vi "Ann_int.vi"(0 "Data":dbl[](array[numeric]), 1 "Loss Function":enum16{"MSE", "MAE"}(ring), 2 "Regularization":T1, 5 "Target":dbl format="%#_13g", 7 "Training?":bool, 9 "Parameters":T3, 13 "Adam Data In":T2) -> (4 "Output":dbl, 6 "Error":dbl, 10 "Adjusted Parameters":T3, 14 "Adam Data Out":T2)   [LabVIEW 2018]
uses:
  Adam_data.ctl
  Globals.vi
  Layer.vi
  Layer1d.vi
panel:
  out "Error Codes":i32[](array[numeric])
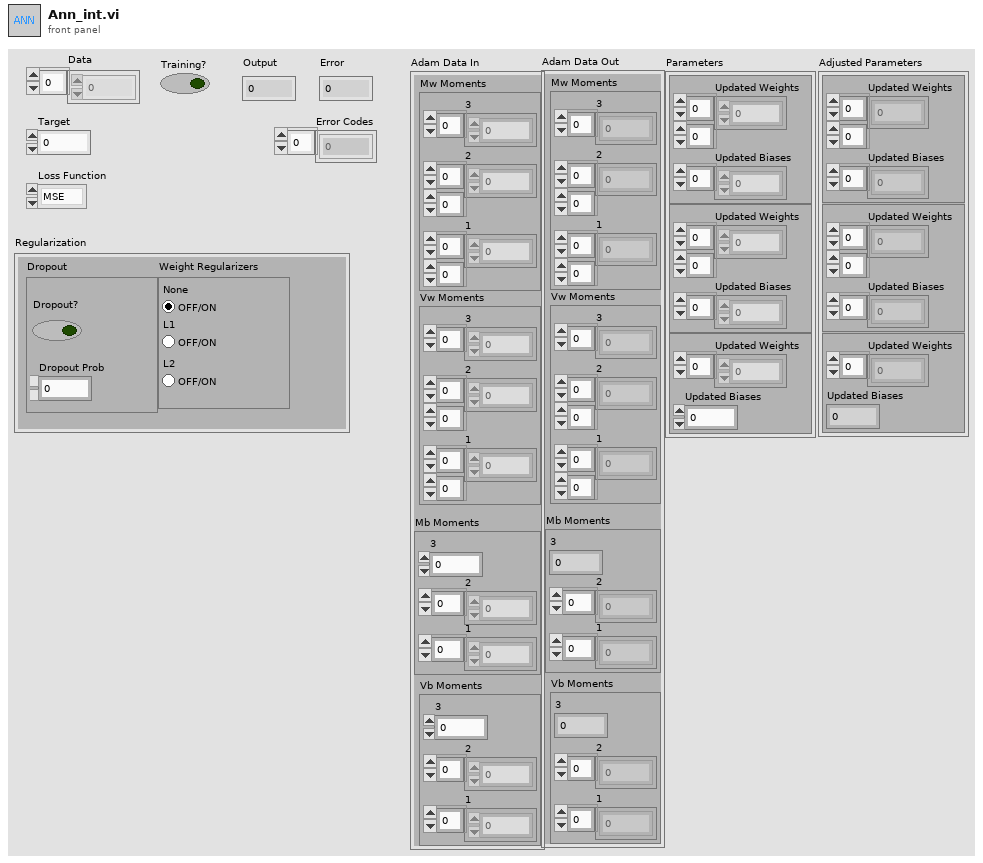
[diagram p1: front panel]
types:
  T1 = cluster{"Dropout":cluster{"Dropout?":bool, "Dropout Prob":dbl}, "Weight Regularizers":enum32{"None", "L1", "L2"}}
  T2 = typedef "Adam_data.ctl" = cluster{"Mw Moments":cluster{"3 ":dbl[], "2":dbl[][], "1":dbl[][]}, "Vw Moments":cluster{"3":dbl[], "2":dbl[][], "1":dbl[][]}, "Mb Moments":cluster{"3":dbl, "2":dbl[], "1":dbl[]}, "Vb Moments":cluster{"3":dbl, "2":dbl[], "1":dbl[]}}
  T3 = cluster{cluster{"Updated Weights":dbl[][], "Updated Biases":dbl[]}, cluster{"Updated Weights":dbl[][], "Updated Biases":dbl[]}, cluster{"Updated Weights":dbl[], "Updated Biases":dbl}}
  T4 = cluster{"Updated Weights":dbl[][], "Updated Biases":dbl[]}
  T5 = cluster{"Updated Weights":dbl[], "Updated Biases":dbl}
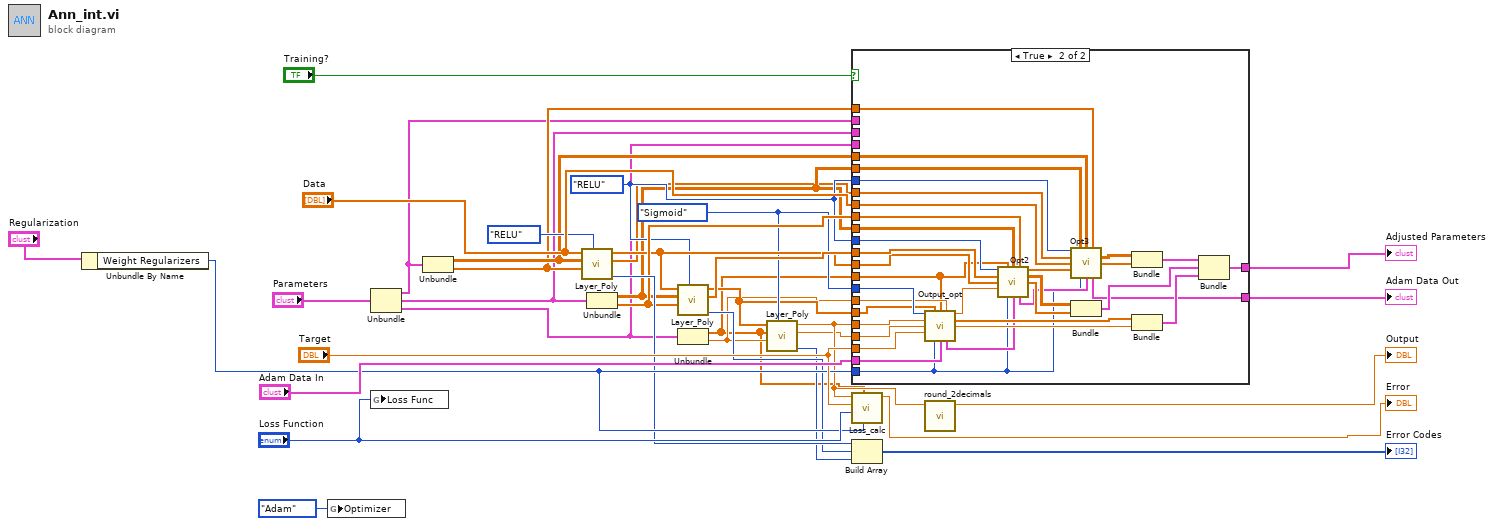
[diagram p0: block diagram]
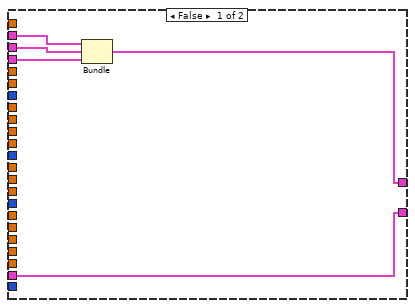
[diagram p2: hidden frame]
diagram:
  w9 = enum32{"Sigmoid", "RELU", "Tanh", "Leaky RELU"}."Sigmoid" ("Activation Function")
  w14 = enum32{"Sigmoid", "RELU", "Tanh", "Leaky RELU"}."RELU" ("Activation Function")
  n1 = Unbundle By Name("Regularization") -> ("Weight Regularizers"=w22:enum32{"None", "L1", "L2"})
  n2 = global write "Globals.vi" "Optimizer"(enum16{"Adagrad", "Adadelta", "Adam"}."Adam" ("Optimizer")) -> ()
  n3 = Unbundle("Parameters") -> (w5:T4, w4:T4, w3:T5)
  n4 = global write "Globals.vi" "Loss Func"("Loss Function") -> ()
  n5 = Unbundle(w5) -> ("Updated Weights"=w12:dbl[][], "Updated Biases"=w11:dbl[])
  n6 = call-poly "Layer_Poly.vi"("Activation Function"=enum32{"Sigmoid", "RELU", "Tanh", "Leaky RELU"}."RELU", "Biases"=w11, "Weights"=w12, "Data"="Data") -> ("Error"=w21:i32, "Net Activation"=w10:dbl[], "Output"=w15:dbl[])  [unwired: 5 in]
  n7 = Unbundle(w4) -> ("Updated Weights"=w13:dbl[][], "Updated Biases"=w17:dbl[])
  n8 = call-poly "Layer_Poly.vi"("Activation Function"=w14, "Biases"=w17, "Weights"=w13, "Data"=w15) -> ("Error"=w20:i32, "Net Activation"=w16:dbl[], "Output"=w8:dbl[])  [unwired: 5 in]
  n9 = Unbundle(w3) -> ("Updated Weights"=w1:dbl[], "Updated Biases"=w2:dbl)
  n10 = call-poly "Layer_Poly.vi"("Activation Function"=w9, "Biases"=w2, "Weights"=w1, "Data"=w8) -> ("Error"=w19:i32, "Net Activation"=w6:dbl, "Output"=w7:dbl)  [unwired: 5 in]
  n11 = case shown="True" "Training?" {
    tunnel: w14 -> [_ w75]
    tunnel: w13 -> [_ w74]
    tunnel: w17 -> [_ w73]
    tunnel: w16 -> [_ w72]
    tunnel: w15 -> [_ w71]
    tunnel: w14 -> [_ w70]
    tunnel: w13 -> [_ w69]
    tunnel: w12 -> [_ w68]
    tunnel: w11 -> [_ w67]
    tunnel: w10 -> [_ w66]
    tunnel: "Data" -> [_ w65]
    tunnel: w9 -> [_ w63]
    tunnel: w8 -> [_ w62]
    tunnel: w7 -> [_ w61]
    tunnel: w6 -> [_ w60]
    tunnel: "Target" -> [_ w59]
    tunnel: [w37 w44] -> w30
    tunnel: w5 -> [w40 _]
    tunnel: w4 -> [w39 _]
    tunnel: w3 -> [w38 _]
    tunnel: w1 -> [_ w51]
    tunnel: w2 -> [_ w52]
    tunnel: [w36 w43] -> w29
    tunnel: "Adam Data In" -> [w36 w42]
    tunnel: w22 -> [_ w41]
    frame False {
      n12 = Bundle(w40, w39, w38) -> (w37:T3)  [unwired: 1 in]
    }
    frame True {
      n13 = call "Output_opt.vi"("Activation Function"=w63, "Activation l-1"=w62, "Weights"=w51, "Biases"=w52, "Activation"=w61, "Net Output"=w60, "Target"=w59, "Weight Regularizers"=w41, "Adam Data In"=w42) -> ("Delta"=w58:dbl, "Updated Weights"=w55:dbl[], "Updated Biases"=w54:dbl, "Adam Data Out"=w46:T2)  [unwired: 3 in]
      n14 = call "Opt2.vi"("Activation Function"=w75, "Weights l+1"=w51, "Weights"=w74, "Biases"=w73, "Net Output"=w72, "Activations l-1"=w71, "Delta l+1"=w58, "Weight Regularizers"=w41, "Adam Data In"=w46) -> ("Delta l"=w64:dbl[], "Updated Weights"=w50:dbl[][], "Updated Biases"=w49:dbl[], "Adam Data Out"=w45:T2)  [unwired: 3 in]
      n15 = call "Opt3.vi"("Activation Function"=w70, "Weights l+1"=w69, "Weights"=w68, "Biases"=w67, "Net Output"=w66, "Activations l-1"=w65, "Delta l+1"=w64, "Weight Regularizers"=w41, "Adam Data In"=w45) -> ("Updated Weights"=w48:dbl[][], "Updated Biases"=w47:dbl[], "Adam Data Out"=w43:T2)  [unwired: 4 in]
      n16 = Bundle("Updated Weights"=w50, "Updated Biases"=w49) -> (w57:T4)  [unwired: 1 in]
      n17 = Bundle("Updated Weights"=w48, "Updated Biases"=w47) -> (w56:T4)  [unwired: 1 in]
      n18 = Bundle("Updated Weights"=w55, "Updated Biases"=w54) -> (w53:T5)  [unwired: 1 in]
      n19 = Bundle(w56, w57, w53) -> (w44:T3)  [unwired: 1 in]
    }
  }
  "Adjusted Parameters" <- w30
  "Adam Data Out" <- w29
  n20 = call "Loss_calc.vi"("Weight Regularizers"=w22, "Weights"=w1, "Loss Type"="Loss Function", "Target"="Target", "Data"=w7) -> ("Loss"=→"Error":dbl)  [unwired: 6 in]
  n21 = Build Array(w21, w20, w19) -> (→"Error Codes":i32[])
  n22 = call "round_2decimals.vi"("Number"=w7) -> ("Rounded Number"=→"Output":dbl)  [unwired: 10 in]
